vi "Get Serial Numbers.vi"(8 "Serial Number":string, 9 "Pass/Fail":bool, 10 "FTT Reject in":u32, 11 "Refnum in":T1) -> (1 "Array":string[](array[string]), 2 "FTT Reject out":u32, 3 "Refnum out":T1)   [LabVIEW 2018]
uses:
  <vilib>/Utility/config.llb/Config Data RefNum.ctl
  <vilib>/Utility/config.llb/Read Key (String).vi
  <vilib>/Utility/config.llb/NI_LVConfig.lvlib
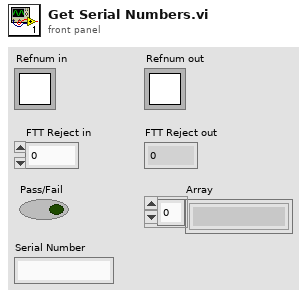
[diagram p1: front panel]
types:
  T1 = typedef "NI_LVConfig.lvlib/Config Data RefNum.ctl" = refnum<k1>
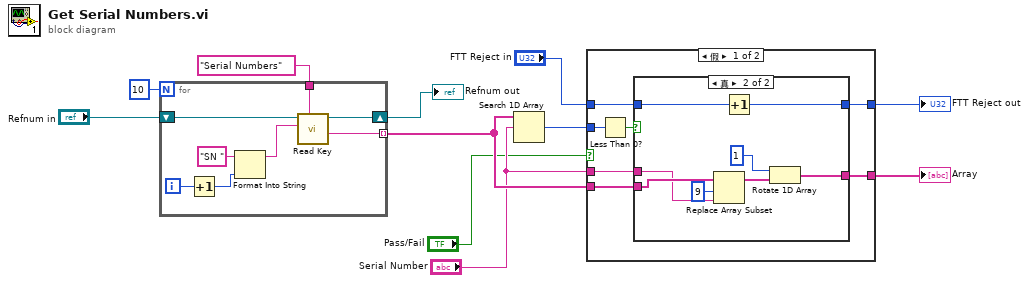
[diagram p0: block diagram]
diagram:
  n1 = for {
    N: 10 ("Total Hours per Shift") -> [_]
    tunnel: "Serial Numbers" ("Shift") -> [w19]
    shift-right: [w13] -> w11
    shift-left: "Refnum in" -> [w14]
    tunnel: [w12] -> w9 mode=indexing
    i -> [w15]
    n2 = Increment(x=w15) -> (x+1=w16:i32)
    n3 = Format Into String(initial string="SN ", w16) -> (resulting string=w18:string)  [unwired: 2 in, 1 out]
    n4 = call-poly <vilib>:"Read Key.vi"("section"=w19, "key"=w18, "refnum"=w14) -> ("value"=w12:string, "refnum out"=w13:T1)  [unwired: 5 in, 2 out]
  }
  "Refnum out" <- w11
  n5 = Search 1D Array(1D array=w9, element="Serial Number") -> (index of element=w7:i32)  [unwired: 1 in]
  n6 = case shown="假" "Pass/Fail" {
    tunnel: "FTT Reject in" -> [w24 w38]
    tunnel: "Serial Number" -> [w21 _]
    tunnel: w9 -> [w22 w37]
    tunnel: [w23 w38] -> w10
    tunnel: w7 -> [w25 _]
    tunnel: [w20 w37] -> w8
    frame False {
      n7 = Less Than 0?(x=w25) -> (x < 0?=w26:bool)
      n8 = case shown="真" w26 {
        tunnel: w24 -> [w28 w36]
        tunnel: [w28 w35] -> w23
        tunnel: w22 -> [w27 w31]
        tunnel: w21 -> [_ w30]
        tunnel: [w27 w29] -> w20
        frame False {
        }
        frame True {
          n9 = Replace Array Subset(array=w31, new element=w30, index=9) -> (w33:string[])
          n10 = Increment(x=w36) -> (x+1=w35:u32)
          n11 = Rotate 1D Array(1:w33, 2:1 ("n")) -> (0:w29:string[])
        }
      }
    }
    frame True {
    }
  }
  "FTT Reject out" <- w10
  "Array" <- w8
